vi "test ws standalone.vi"() -> ()   [LabVIEW 2016]
uses:
  websocket/standalone server/websocket standalone server.lvclass
  websocket/standalone server/websocket message type.ctl
  websocket/standalone server/websocket data packet.ctl
  websocket/standalone server/websocket connection parameters.ctl
panel:
  out "lengthr":i32
  out "lengths":i32
  in  "send txt":bool
  in  "DATA to send":string
  out "conn idx":i32
  out "data":string
  out "message type":T1
  in  "parameters":T2={"port"=80, "supported subprotocols"=[]}
  in  "stop":bool
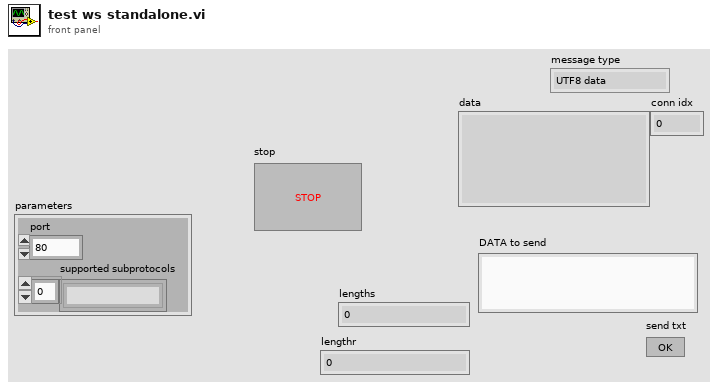
[diagram p1: front panel]
types:
  T1 = typedef "websocket standalone server.lvclass/websocket message type.ctl" = enum16{"UTF8 data", "binary data", "close", "ping", "pong"}
  T2 = typedef "websocket standalone server.lvclass/websocket connection parameters.ctl" = cluster{"port":u16, "supported subprotocols":string[]}
  T3 = typedef "websocket standalone server.lvclass/websocket data packet.ctl" = cluster{"message type":T1, "data":string}
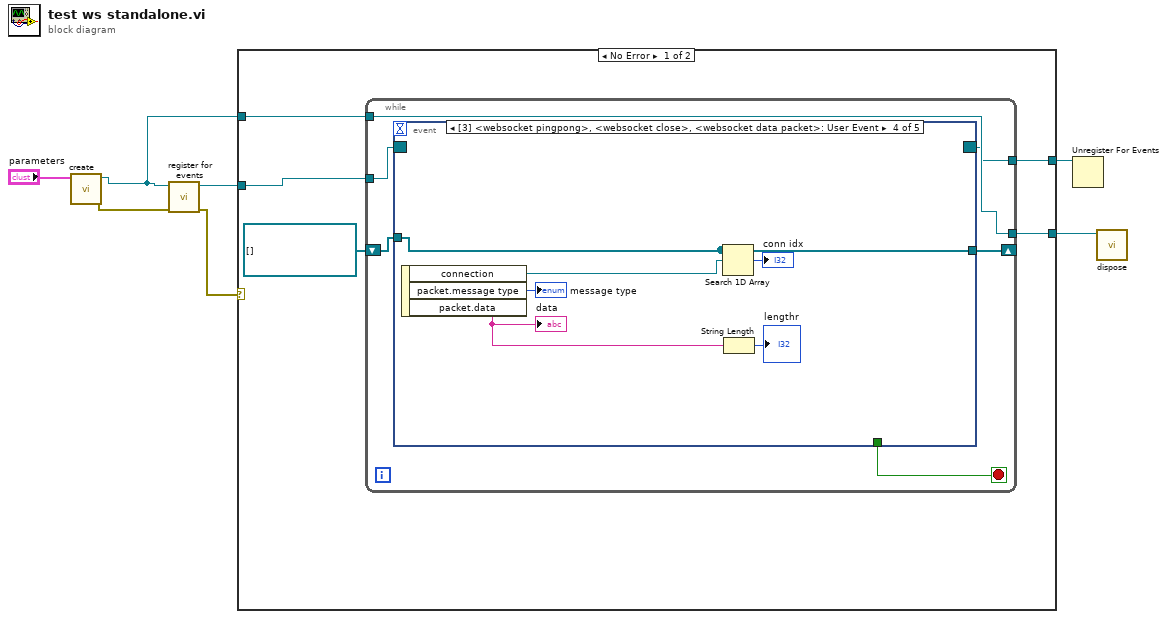
[diagram p0: block diagram]
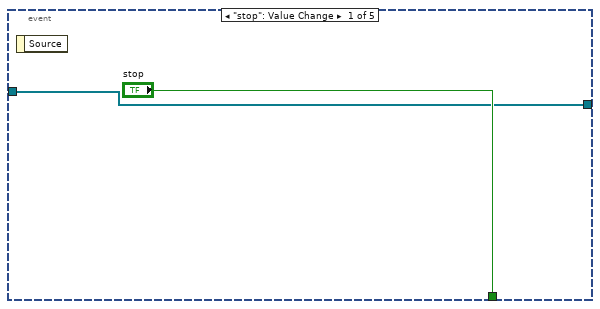
[diagram p2: hidden frame]
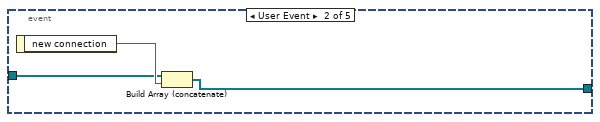
[diagram p3: hidden frame]
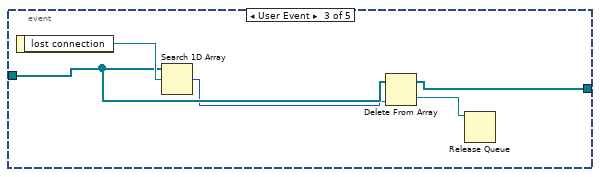
[diagram p4: hidden frame]
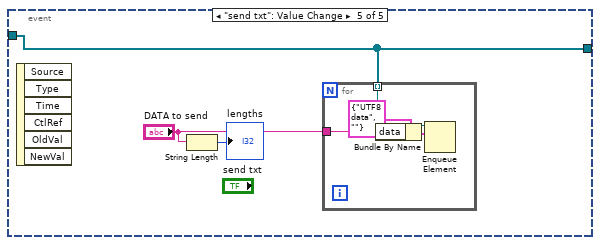
[diagram p5: hidden frame]
diagram:
  n1 = call "create.vi"("parameters"="parameters") -> ("error out"=w7:errorcluster, "websocket standalone server out"=w6:refnum<class "websocket standalone server.lvclass">)  [unwired: 9 in]
  n2 = call "register for events.vi"("error in"=w7, "websocket standalone server in"=w6) -> ("error out"=w1:errorcluster, "event registration"=w4:refnum<event-registration>)  [unwired: 8 in]
  n3 = case shown="No Error" w1 {
    tunnel: w6 -> [w12 w42]
    tunnel: [w11 w42] -> w5
    tunnel: w4 -> [w10 w43]
    tunnel: [w9 w43] -> w3
    frame No Error {
      n4 = while {
        tunnel: w12 -> [w17]
        tunnel: [w17] -> w11
        tunnel: w10 -> [w16]
        tunnel: [w15] -> w9
        shift-right: [w14] -> _
        shift-left: refnum<queue>[] [] -> [w13]
        stop <- w18 stop-if-true
        n5 = event shown="[3] <websocket pingpong>, <websocket close>, <websocket data packet>: User Event" {
          selector: w16 -> [_ _ _ _ _]
          dyn-events: [_ _ _ _ _] -> w15
          timeout: _ -> [_ _ _ _ _]
          tunnel: ["stop" _ _ _ _] -> w18
          tunnel: [w19 w22 w25 w33 w37] -> w14
          tunnel: w13 -> [w19 w21 w27 w33 w37]
          event "stop": Value Change {
            n6 = event-data() -> ()  [unwired: 1 in, 1 out]
          }
          event User Event {
            n7 = event-data() -> ("new connection"=w23:refnum<queue>)  [unwired: 1 in]
            n8 = Build Array (concatenate)(w21, w23) -> (w22:refnum<queue>[])
          }
          event User Event {
            n9 = event-data() -> ("lost connection"=w28:refnum<queue>)  [unwired: 1 in]
            n10 = Search 1D Array(1D array=w27, element=w28) -> (index of element=w26:i32)  [unwired: 1 in]
            n11 = Delete From Array(array=w27, index=w26) -> (deleted portion=w24:refnum<queue>, array with subset deleted=w25:refnum<queue>[])  [unwired: 1 in]
            n12 = Release Queue(queue=w24) -> ()  [unwired: 2 in, 3 out]
          }
          event User Event {
            n13 = event-data() -> ("connection"=w32:refnum<queue>, "packet.message type"=→"message type":T1, "packet.data"=w29:string)  [unwired: 1 in]
            "data" <- w29
            n14 = Search 1D Array(1D array=w33, element=w32) -> (index of element=→"conn idx":i32)  [unwired: 1 in]
            n15 = String Length(string=w29) -> (length=→"lengthr":i32)
          }
          event "send txt": Value Change {
            n16 = event-data() -> ()  [unwired: 1 in, 6 out]
            n17 = String Length(string="DATA to send") -> (length=→"lengths":i32)
            n18 = for {
              tunnel: w37 -> [w41] mode=indexing
              tunnel: "DATA to send" -> [w38]
              n19 = Bundle By Name(cluster=T3 {"message type"=enum."UTF8 data", "data"=""} ("element"), "data"=w38) -> (w39:T3)
              n20 = Enqueue Element(queue=w41, element=w39) -> ()  [unwired: 2 in, 3 out]
            }
          }
        }
      }
    }
    frame Error {
    }
  }
  n21 = Unregister For Events(event registration refnum=w3) -> ()  [unwired: 1 in, 1 out]
  n22 = call "dispose.vi"("websocket standalone server in"=w5) -> ()  [unwired: 10 in, 1 out]
